vi "Test 2 Reveal Second Set of Cubes.vi"(8 "error in (no error)":errorcluster, 11 "Test Case In":refnum<class "Game Test.lvclass">) -> (0 "error out":errorcluster, 3 "Test Case Out":refnum<class "Game Test.lvclass">)   [LabVIEW 2020, in "Game Test.lvclass"]
uses:
  Game Test.lvclass
  C:/Program Files (x86)/National Instruments/LabVIEW 2020/vi.lib/Astemes/LUnit/Test Case.lvclass
  Bag/Cubes.ctl
  <vilib>/Astemes/LUnit/Test Case.lvclass/Test Case.ctl
  4993e8ee-a06a-463a-9684-69129f64d5ce.vi
  <vilib>/Astemes/LUnit/Append Pass Result.vi
  <vilib>/Astemes/LUnit/Append Fail Result.vi
  <vilib>/Astemes/LUnit/Describe Comparison.vi
  <vilib>/Astemes/LUnit/Compare Variants.vi
  <vilib>/Astemes/LUnit/Variant to string.vi
  <vilib>/Utility/Data Type/Get Type Information.vi
  <vilib>/Utility/LVClass/Get LV Class Name.vi
  Bag/Bag.lvclass
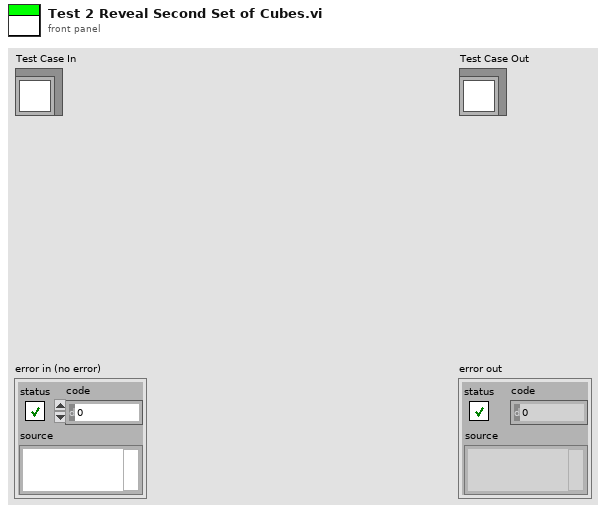
[diagram p1: front panel]
types:
  T1 = typedef "Bag.lvclass/Cubes.ctl" = cluster{"Red":i32, "Green":i32, "Blue":i32}
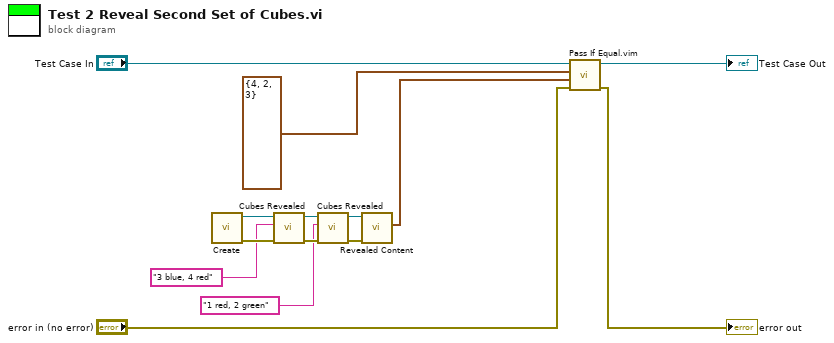
[diagram p0: block diagram]
diagram:
  n1 = call "Create.vi"() -> ("error out"=w9:errorcluster, "Bag"=w10:refnum<class "Bag.lvclass">)  [unwired: 10 in]
  n2 = call "Cubes Revealed.vi"("error in (no error)"=w9, "Set"="3 blue, 4 red", "Bag in"=w10) -> ("error out"=w7:errorcluster, "Bag out"=w3:refnum<class "Bag.lvclass">)  [unwired: 7 in]
  n3 = call "Cubes Revealed.vi"("error in (no error)"=w7, "Set"="1 red, 2 green", "Bag in"=w3) -> ("error out"=w4:errorcluster, "Bag out"=w2:refnum<class "Bag.lvclass">)  [unwired: 7 in]
  n4 = call "Revealed Content.vi"("error in (no error)"=w4, "Bag in"=w2) -> ("Cubes"=w6:T1)  [unwired: 7 in, 2 out]
  n5 = call "Pass If Equal.vim"("error in (no error)"="error in (no error)", "Actual"=w6, "Expected"=T1 {"Red"=4, "Green"=2, "Blue"=3} ("Cubes"), "LUnit Test Case In"="Test Case In") -> ("error out"=→"error out":errorcluster, "LUnit Test Case Out"=→"Test Case Out":refnum<class "Game Test.lvclass">)  [unwired: 6 in]
